vi "build.volume.data.vi"() -> ()   [LabVIEW 2024]
panel:
  in  "characters":string[](array[string])
  out "found":i32
  out "current file":string
  out "volumes":T1(array[cluster])
  in  "team":string[](array[string])
  in  "Threshold":dbl
  in  "first letter":string
  in  "Folder Path":path
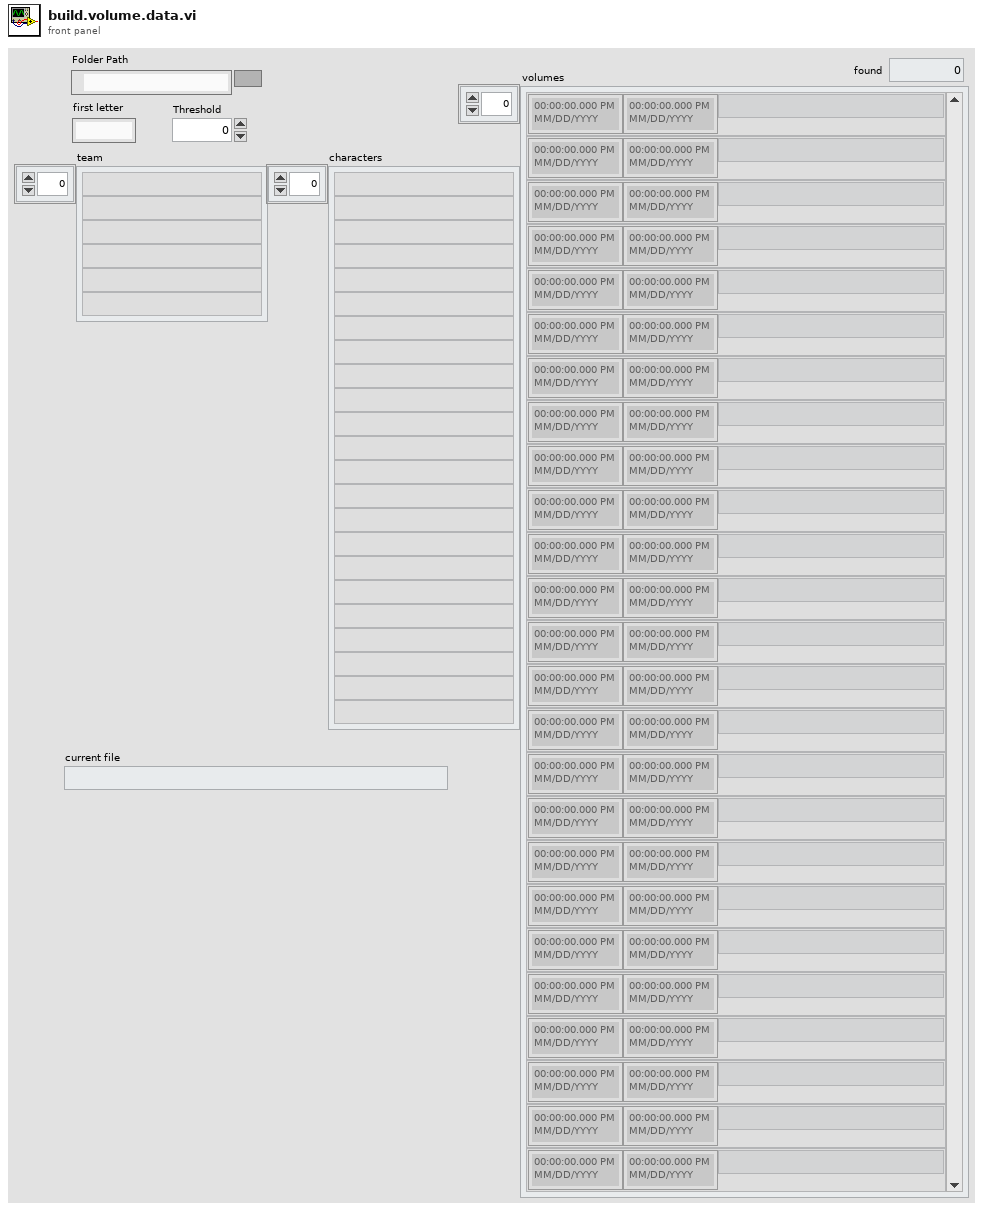
[diagram p1: front panel]
types:
  T1 = cluster{"start date":timestamp, "end date":timestamp, "sortable_name":string}[]
  T2 = typedef "comicvine_issue.generic_credit.ctl" = cluster{"id":i32, "name":string}
  T3 = cluster{"start date":timestamp, "end date":timestamp, "sortable_name":string}
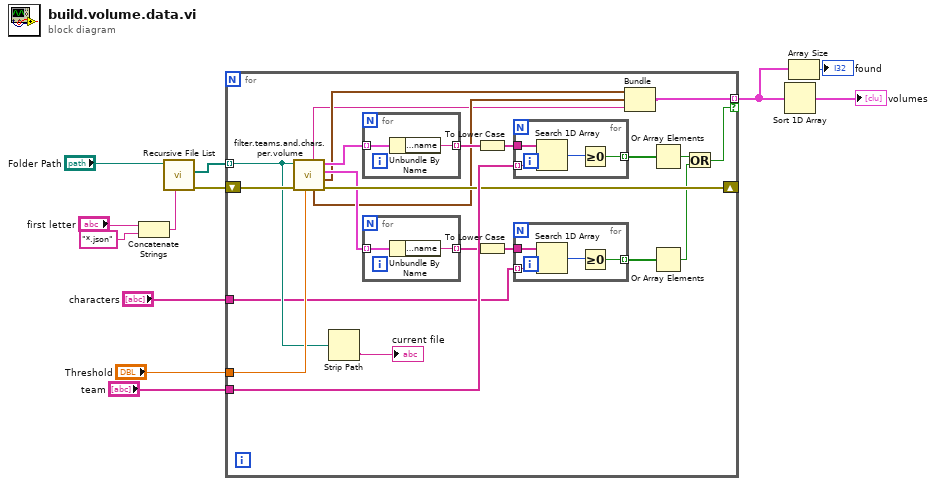
[diagram p0: block diagram]
diagram:
  n1 = Concatenate Strings("first letter", "*.json" ("string")) -> (w9:string)
  n2 = call <vilib>:"Recursive File List.vi"("pattern"=w9, "Folder Path"="Folder Path") -> ("error out"=w8:errorcluster, "All Files in Dir"=w7:path[])  [unwired: 5 in, 3 out]
  n3 = for {
    tunnel: w7 -> [w25] mode=indexing
    tunnel: "Threshold" -> [w31]
    tunnel: "team" -> [w29]
    shift-right: [w28] -> _
    shift-left: w8 -> [w34]
    tunnel: [w27] -> w4 mode=indexing if=w18
    tunnel: "characters" -> [w16]
    n4 = call "filter.teams.and.chars.per.volume.vi"("Threshold"=w31, "error in"=w34, "volume json"=w25) -> ("error out"=w28:errorcluster, "start date"=w15:timestamp, "Chars Ranked"=w20:cluster{"size":i32, "character_credit":T2}[], "Teams Ranked"=w33:cluster{"size":i32, "character_credit":T2}[], "end date"=w14:timestamp, "sortable_name"=w13:string)  [unwired: 3 in]
    n5 = Strip Path(path=w25) -> (name=→"current file":string)  [unwired: 1 out]
    n6 = for {
      tunnel: w33 -> [w46] mode=indexing
      tunnel: [w45] -> w32 mode=indexing
      n7 = Unbundle By Name(w46) -> ("character_credit.name"=w45:string)
    }
    n8 = for {
      tunnel: w20 -> [w40] mode=indexing
      tunnel: [w39] -> w21 mode=indexing
      n9 = Unbundle By Name(w40) -> ("character_credit.name"=w39:string)
    }
    n10 = To Lower Case(string=w32) -> (all lower case string=w30:string[])
    n11 = To Lower Case(string=w21) -> (all lower case string=w22:string[])
    n12 = for {
      tunnel: w30 -> [w44]
      tunnel: w29 -> [w43] mode=indexing
      tunnel: [w41] -> w26 mode=indexing
      n13 = Search 1D Array(1D array=w44, element=w43) -> (index of element=w42:i32)  [unwired: 1 in]
      n14 = Greater Or Equal To 0?(x=w42) -> (x >= 0?=w41:bool)
    }
    n15 = for {
      tunnel: w22 -> [w38]
      tunnel: w16 -> [w37] mode=indexing
      tunnel: [w35] -> w23 mode=indexing
      n16 = Search 1D Array(1D array=w38, element=w37) -> (index of element=w36:i32)  [unwired: 1 in]
      n17 = Greater Or Equal To 0?(x=w36) -> (x >= 0?=w35:bool)
    }
    n18 = Bundle("start date"=w15, "end date"=w14, "sortable_name"=w13) -> (w27:T3)  [unwired: 1 in]
    n19 = Or Array Elements(Boolean array=w26) -> (logical OR=w19:bool)
    n20 = Or Array Elements(Boolean array=w23) -> (logical OR=w17:bool)
    n21 = Or(x=w19, y=w17) -> (x .or. y?=w18:bool)
  }
  n22 = Sort 1D Array(array=w4) -> (sorted array=→"volumes":T1)
  n23 = Array Size(array=w4) -> (size(s)=→"found":i32)
